vi "GPIO.vi"() -> ()   [LabVIEW 2010]
uses:
  libdaqVI.lvlib
panel:
  out "采集卡状态":bool
  out "GPIOOUT IO数量":u8
  out "GPIOIN IO数量":u8
  out "DI5":bool
  out "DI4":bool
  out "DI3":bool
  out "DI2":bool
  out "DI1":bool
  out "DI0":bool
  in  "DO5":bool
  in  "DO4":bool
  in  "DO3":bool
  in  "DO2":bool
  in  "DO1":bool
  in  "DO0":bool
  in  "?":bool
  in  "GPIO操作函数类型选择":T1(radio)
  out "设备名称":string
  out "设备数量":i32
  # "GPIO模块操作演示程序"
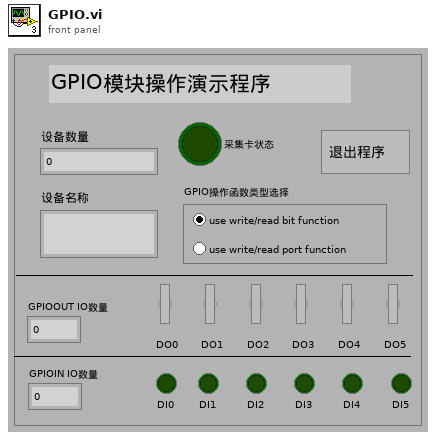
[diagram p1: front panel]
types:
  T1 = enum32{"use write/read bit function", "use write/read port function"}
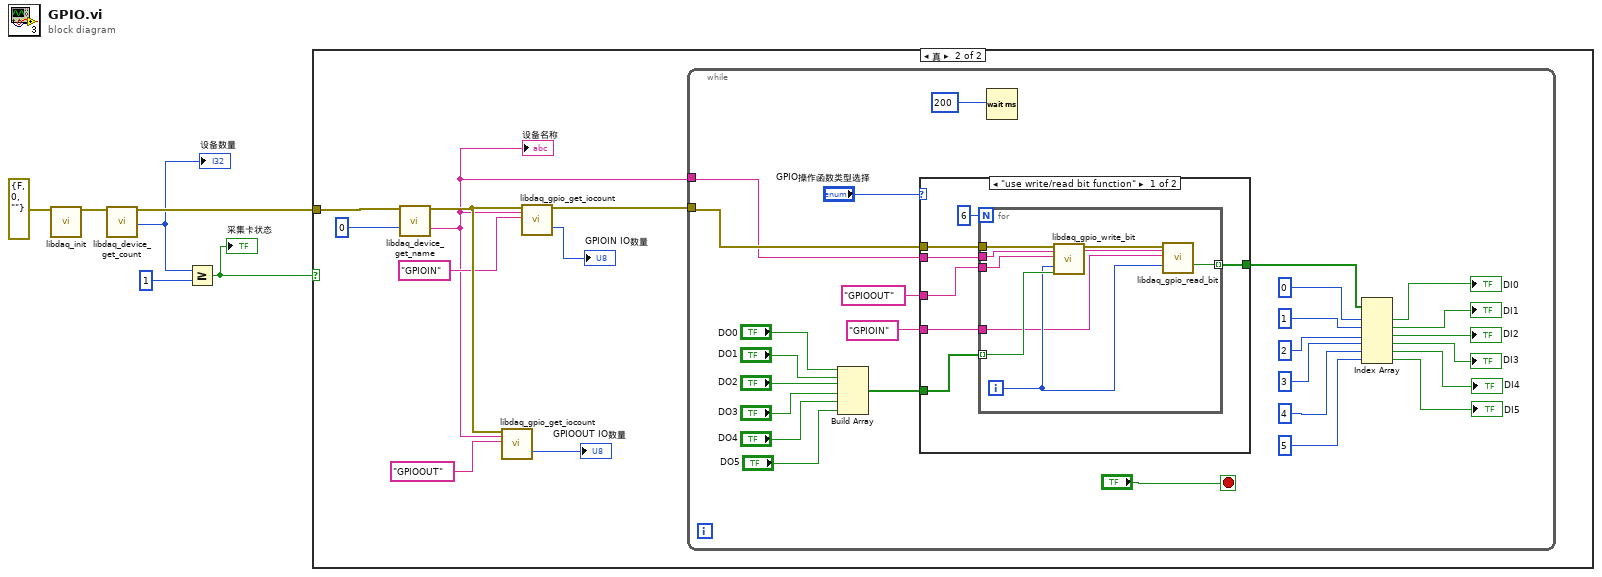
[diagram p0: block diagram]
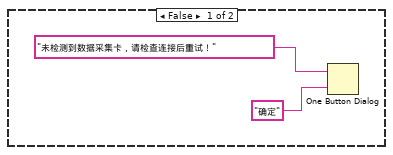
[diagram p2: hidden frame]
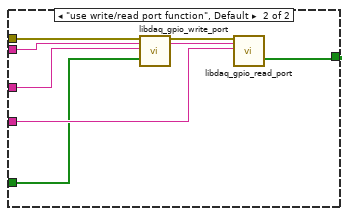
[diagram p3: hidden frame]
diagram:
  n1 = call "libdaq_init.vi"("error in (no error)"=errorcluster {"status"=FALSE, "code"=0, "source"=""}) -> ("error out"=w6:errorcluster)  [unwired: 18 in]
  n2 = call "libdaq_device_get_count.vi"("error in (no error)"=w6) -> ("error out"=w4:errorcluster, "device_count"=w1:i32)  [unwired: 17 in]
  "设备数量" <- w1
  n3 = Greater Or Equal?(x=w1, y=u32 1 ("name length")) -> (x >= y?=w2:bool)
  "采集卡状态" <- w2
  n4 = case shown="真" w2 {
    tunnel: w4 -> [_ w17]
    frame False {
      n5 = One Button Dialog(message="未检测到数据采集卡，请检查连接后重试！" ("消息"), button name ("OK")="确定" ("按钮名称（“确定”）")) -> ()  [unwired: 1 out]
    }
    frame True {
      n6 = call "libdaq_device_get_name.vi"("error in (no error)"=w17, "device_index"=u32 0 ("name length")) -> ("error out"=w13:errorcluster, "device_name"=w9:string)  [unwired: 16 in]
      "设备名称" <- w9
      n7 = call "libdaq_gpio_get_iocount.vi"("error in (no error)"=w13, "device_name"=w9, "module_name"="GPIOOUT") -> ("iocount"=→"GPIOOUT IO数量":u8)  [unwired: 13 in, 3 out]
      n8 = call "libdaq_gpio_get_iocount.vi"("error in (no error)"=w13, "device_name"=w9, "module_name"="GPIOIN") -> ("error out"=w11:errorcluster, "iocount"=→"GPIOIN IO数量":u8)  [unwired: 13 in, 2 out]
      n9 = while {
        tunnel: w11 -> [w41]
        tunnel: w9 -> [w40]
        stop <- "?" stop-if-true
        n10 = Build Array("DO0", "DO1", "DO2", "DO3", "DO4", "DO5") -> (w39:bool[])
        n11 = case shown="\"use write/read bit function\"" "GPIO操作函数类型选择" {
          tunnel: w41 -> [w50 w66]
          tunnel: w40 -> [w49 w65]
          tunnel: w39 -> [w46 w62]
          tunnel: "GPIOIN" -> [w48 w63]
          tunnel: "GPIOOUT" -> [w45 w64]
          tunnel: [w47 w61] -> w24
          frame "use write/read bit function" {
            n12 = for {
              N: 6 -> [_]
              tunnel: w50 -> [w60]
              tunnel: w49 -> [w58]
              tunnel: w46 -> [w59] mode=indexing
              tunnel: [w54] -> w47 mode=indexing
              tunnel: w48 -> [w53]
              tunnel: w45 -> [w52]
              i -> [w55]
              n13 = call "libdaq_gpio_write_bit.vi"("error in (no error)"=w60, "device_name"=w58, "module_name"=w52, "ioIndex"=w55, "BitVal"=w59) -> ("error out"=w57:errorcluster, "device_name"=w56:string)  [unwired: 12 in, 1 out]
              n14 = call "libdaq_gpio_read_bit.vi"("error in (no error)"=w57, "device_name"=w56, "module_name"=w53, "ioIndex"=w55) -> ("BitVal"=w54:bool)  [unwired: 12 in, 3 out]
            }
          }
          frame "use write/read port function", Default {
            n15 = call "libdaq_gpio_write_port.vi"("error in (no error)"=w66, "device_name"=w65, "module_name"=w64, "portval"=w62) -> ("error out"=w67:errorcluster)  [unwired: 13 in, 2 out]
            n16 = call "libdaq_gpio_read_port.vi"("error in (no error)"=w67, "device_name"=w65, "module_name"=w63) -> ("portval"=w61:bool[])  [unwired: 13 in, 3 out]
          }
        }
        n17 = Wait (ms)(milliseconds to wait=200) -> ()  [unwired: 1 out]
        n18 = Index Array(array=w24, index #1=0, index #2=1, index #3=2, index #4=3, index #5=4, index #6=5) -> (element #1=→"DI0":bool, element #2=→"DI1":bool, element #3=→"DI2":bool, element #4=→"DI3":bool, element #5=→"DI4":bool, element #6=→"DI5":bool)
      }
    }
  }
